vi "qTIM.vi"(0 "System no.":i32=1 min=1 max=4 step=1, 5 "error in":errorcluster) -> (14 "System time":i32, 15 "Time (Float)":dbl, 19 "error out":errorcluster)   [LabVIEW 2020]
doc: "GCS 1.0: Returns controller system time (integer). GCS 2.0 or higher: Reports the number of milliseconds (float) since start-up or last TIM command (if supported).\n\nC-702: Reports system time as number of servo-loop counts (independent of servo-control mode) since firmware program start; duration of one loop is 100 µs.\nC-848: Reports system time as number of servo-loop counts (independent of servo-control mode) since firmware program start; duration of one loop is 400 µs.\nC-867, C-884: Reports the number of milliseconds (float) since start-up or last TIM command. System time is not valid. \nC-880: Reports system time as number of servo-loop counts (independent of servo-control mode) since firmware program start; duration of one loop is 400 µs."
panel:
  # "Returns controller system time."
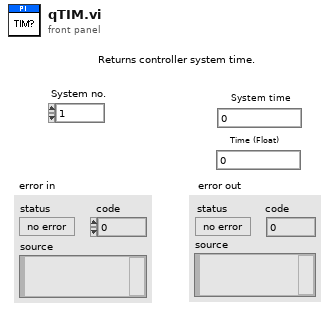
[diagram p1: front panel]
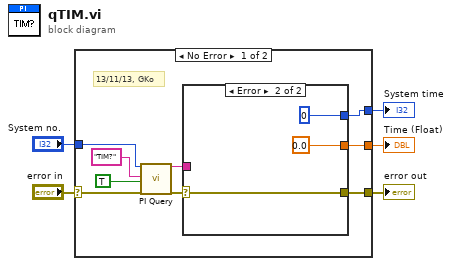
[diagram p0: block diagram]
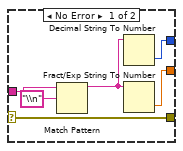
[diagram p2: hidden frame]
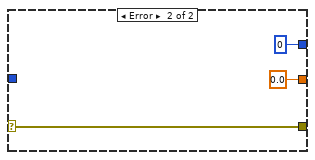
[diagram p3: hidden frame]
diagram:
  n1 = case shown="No Error" "error in" {
    selector: "error in" -> [w6 w26]
    tunnel: [w14 0] -> w5
    tunnel: "System no." -> [w12 _]
    tunnel: [w10 0.0] -> w3
    tunnel: [w7 w26] -> w2
    frame No Error {
      # "13/11/13, GKo"
      n2 = call "PI Query.vi"("System no."=w12, "String to send"="TIM?", "Attach termination char.?"=TRUE ("Attach Linefeed?"), "error in"=w6) -> ("String read"=w9:string, "error out"=w8:errorcluster)  [unwired: 3 in, 11 out]
      n3 = case shown="Error" w8 {
        selector: w8 -> [w15 w21]
        tunnel: w9 -> [w19 _]
        tunnel: [w20 0] -> w14
        tunnel: [w16 0.0] -> w10
        tunnel: [w15 w21] -> w7
        frame No Error {
          n4 = Match Pattern(string=w19, regular expression="\\n") -> (before substring=w17:string)  [unwired: 4 out]
          n5 = Decimal String To Number(string=w17) -> (number=w20:i32)  [unwired: 3 out]
          n6 = Fract/Exp String To Number(string=w17) -> (number=w16:dbl)  [unwired: 4 out]
        }
        frame Error {
        }
      }
    }
    frame Error {
    }
  }
  "error out" <- w2
  "System time" <- w5
  "Time (Float)" <- w3
